vi "attribute_write.vi"(1 "Boolean in":bool, 4 "String in":string, 5 "I64 in":i64, 6 "Repeated Capability":string, 7 "I32 in":i32, 8 "error in":errorcluster, 9 "Double in":dbl, 10 "Attribute ID":string, 11 "VISA resource name":refnum<visa-resource-name>) -> (0 "error out":errorcluster, 3 "VISA resource name out":refnum<visa-resource-name>)   [LabVIEW 2014, in "rszvl_rsidr_core.lvlib"]
uses:
  rszvl_rsidr_core.lvlib
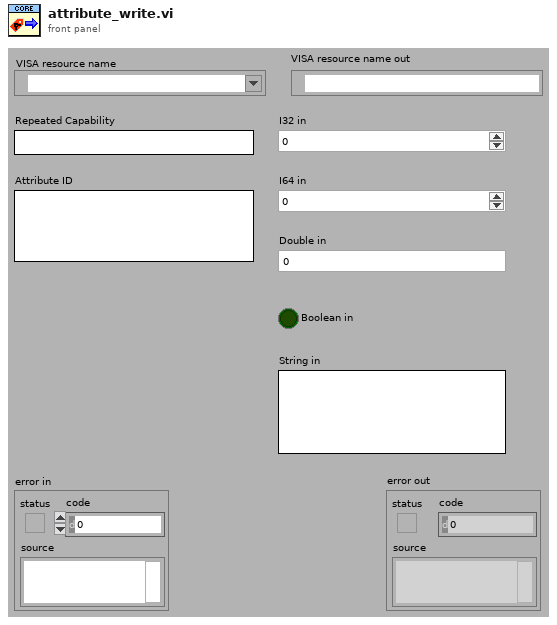
[diagram p1: front panel]
types:
  T1 = typedef "rszvl_rsidr_core.lvlib/type_Attribute.ctl" = cluster{"Identifier":string, "Descriptive name":string, "Data Type":T2, "Command":string, "Access":u16, "Range Table":string, "Read Callback":string, "Write Callback":string, "Range Callback":string, "Check Callback":string, "Rngtable Callback":string, "Coerce Callback":string, "Supported Models":string, "Instrument Options":string, "Repeated Capabilities":string, "Check Status Callback":string, "Index":i32, "Flag: OPC Wait":bool, "Flag: Dont check status":bool, "Flag: Cache Only":bool}
  T2 = typedef "rszvl_rsidr_core.lvlib/type_Attribute_Data_Type.ctl" = enum16{"Integer 32", "Double", "String", "Boolean", "None", "Integer 64"}
  T3 = typedef "rszvl_rsidr_core.lvlib/type_Session_Data.ctl" = cluster{"Instr type":string, "Instr type for err. msg.":string, "Installed Options":string[], "OPC Timeout":i32, "Query Instrument Status":bool, "Check Range":bool, "Check Options":bool, "Add LF to Write":bool, "Simulate":bool, "Logging":bool, "Logging params":variant, "Interface Type":enum16{"Unknown", "GPIB", "VXI", "GPIB_VXI", "ASRL", "PXI", "TCPIP", "USB", "SOCKET"}, "Fast Sweep":i32, "AdditionalFlags":i32, "WaitBeforeWrite":i32, "WaitBeforeRead":i32, "BinDataChunkSize":i64}
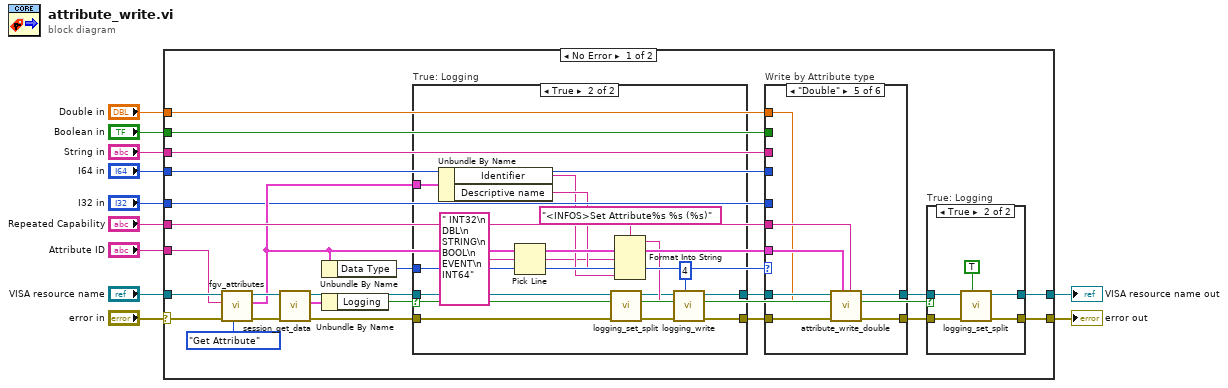
[diagram p0: block diagram]
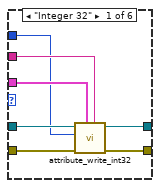
[diagram p4: hidden frame]
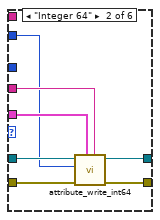
[diagram p5: hidden frame]
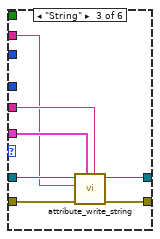
[diagram p6: hidden frame]
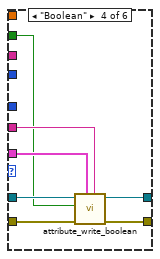
[diagram p7: hidden frame]
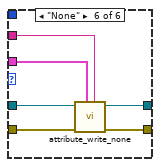
[diagram p8: hidden frame]
diagram:
  n1 = case shown="No Error" "error in" {
    selector: "error in" -> [w21 w100]
    tunnel: "VISA resource name" -> [w32 w101]
    tunnel: "Repeated Capability" -> [w34 _]
    tunnel: [w28 w101] -> w9
    tunnel: [w29 w100] -> w8
    tunnel: "Attribute ID" -> [w19 _]
    tunnel: "I32 in" -> [w16 _]
    tunnel: "I64 in" -> [w15 _]
    tunnel: "String in" -> [w14 _]
    tunnel: "Boolean in" -> [w13 _]
    tunnel: "Double in" -> [w12 _]
    frame No Error {
      n2 = call "fgv_attributes.vi"("Operation"=enum16{"Initialize", "Get Attribute"}."Get Attribute", "error in"=w21, "Attribute ID in"=w19) -> ("error out"=w20:errorcluster, "Attribute out"=w17:T1)  [unwired: 6 in, 1 out]
      n3 = call "session_get_data.vi"("error in"=w20, "VISA resource name"=w32) -> ("error out"=w26:errorcluster, "Session User Data out"=w22:T3, "VISA resource name out"=w25:refnum<visa-resource-name>)  [unwired: 7 in]
      n4 = Unbundle By Name(w17) -> ("Data Type"=w33:T2)
      n5 = Unbundle By Name(w22) -> ("Logging"=w27:bool)
      n6 = case "True: Logging" shown="True" w27 {
        tunnel: w26 -> [w43 w49]
        tunnel: [w43 w45] -> w24
        tunnel: w17 -> [_ w58]
        tunnel: w25 -> [w42 w48]
        tunnel: [w42 w44] -> w23
        tunnel: w33 -> [_ w52]
        frame False {
        }
        frame True {
          n7 = Unbundle By Name(w58) -> ("Identifier"=w55:string, "Descriptive name"=w56:string)
          n8 = Pick Line(multi-line string=" INT32\n DBL\n STRING\n BOOL\n EVENT\n INT64", line index=w52) -> (output string=w51:string)  [unwired: 1 in]
          n9 = call "logging_set_split.vi"("error in"=w49, "VISA resource name"=w48) -> ("error out"=w47:errorcluster, "VISA resource name out"=w46:refnum<visa-resource-name>)  [unwired: 8 in]
          n10 = Format Into String(format string="<INFOS>Set Attribute%s %s (%s)", w51, w56, w55) -> (resulting string=w54:string)  [unwired: 2 in, 1 out]
          n11 = call "logging_write.vi"("Add call chain offset\n(No call chain)"=4 ("Add call chain offset\n(No call chain)"), "error in"=w47, "String to write"=w54, "VISA resource name"=w46) -> ("error out"=w45:errorcluster, "VISA resource name out"=w44:refnum<visa-resource-name>)  [unwired: 6 in]
        }
      }
      n12 = case "Write by Attribute type" shown="\"Double\"" w33 {
        tunnel: w17 -> [w61 w67 w74 w81 w92 w95]
        tunnel: w23 -> [w65 w72 w79 w86 w91 w99]
        tunnel: w24 -> [w64 w71 w78 w85 w88 w94]
        tunnel: w34 -> [w60 w68 w75 w82 w93 w96]
        tunnel: [w63 w70 w77 w84 w89 w98] -> w30
        tunnel: [w62 w69 w76 w83 w90 w97] -> w31
        tunnel: w16 -> [w59 _ _ _ _ _]
        tunnel: w15 -> [_ w66 _ _ _ _]
        tunnel: w14 -> [_ _ w73 _ _ _]
        tunnel: w13 -> [_ _ _ w80 _ _]
        tunnel: w12 -> [_ _ _ _ w87 _]
        frame "Integer 32" {
          n13 = call "attribute_write_int32.vi"("Repeated Capability"=w60, "Attribute"=w61, "error in"=w64, "int32 in"=w59, "VISA resource name"=w65) -> ("error out"=w62:errorcluster, "VISA resource name out"=w63:refnum<visa-resource-name>)  [unwired: 5 in]
        }
        frame "Integer 64" {
          n14 = call "attribute_write_int64.vi"("Repeated Capability"=w68, "Attribute"=w67, "error in"=w71, "int64 in"=w66, "VISA resource name"=w72) -> ("error out"=w69:errorcluster, "VISA resource name out"=w70:refnum<visa-resource-name>)  [unwired: 5 in]
        }
        frame "String" {
          n15 = call "attribute_write_string.vi"("Repeated Capability"=w75, "Attribute"=w74, "error in"=w78, "string in"=w73, "VISA resource name"=w79) -> ("error out"=w76:errorcluster, "VISA resource name out"=w77:refnum<visa-resource-name>)  [unwired: 5 in]
        }
        frame "Boolean" {
          n16 = call "attribute_write_boolean.vi"("Repeated Capability"=w82, "Attribute"=w81, "error in"=w85, "boolean in"=w80, "VISA resource name"=w86) -> ("error out"=w83:errorcluster, "VISA resource name out"=w84:refnum<visa-resource-name>)  [unwired: 5 in]
        }
        frame "Double" {
          n17 = call "attribute_write_double.vi"("Repeated Capability"=w93, "Attribute"=w92, "error in"=w88, "double in"=w87, "VISA resource name"=w91) -> ("error out"=w90:errorcluster, "VISA resource name out"=w89:refnum<visa-resource-name>)  [unwired: 5 in]
        }
        frame "None" {
          n18 = call "attribute_write_none.vi"("Repeated Capability"=w96, "Attribute"=w95, "error in"=w94, "VISA resource name"=w99) -> ("error out"=w97:errorcluster, "VISA resource name out"=w98:refnum<visa-resource-name>)  [unwired: 6 in]
        }
      }
      n19 = case "True: Logging" shown="True" w27 {
        tunnel: w31 -> [w36 w41]
        tunnel: [w36 w39] -> w29
        tunnel: w30 -> [w35 w40]
        tunnel: [w35 w38] -> w28
        frame False {
        }
        frame True {
          n20 = call "logging_set_split.vi"("Evaluate section error (F)"=TRUE, "error in"=w41, "VISA resource name"=w40) -> ("error out"=w39:errorcluster, "VISA resource name out"=w38:refnum<visa-resource-name>)  [unwired: 7 in]
        }
      }
    }
    frame Error {
    }
  }
  "error out" <- w8
  "VISA resource name out" <- w9
